vi "template.created_at.vi"(8 "error in":errorcluster, 11 "Template in":refnum<class "Template.lvclass">) -> (0 "error out":errorcluster, 3 "Template out":refnum<class "Template.lvclass">)   [LabVIEW 2020, in "Template.lvclass"]
doc: "Returns the time the template was created."
uses:
  Template.lvclass
  Template.lvclass/Template.ctl
  client.lvlib
panel:
  out "out_millis out":dbl
  in  "out_millis":dbl
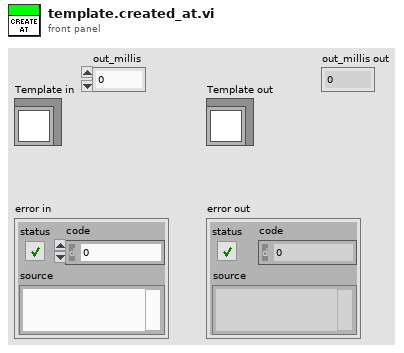
[diagram p1: front panel]
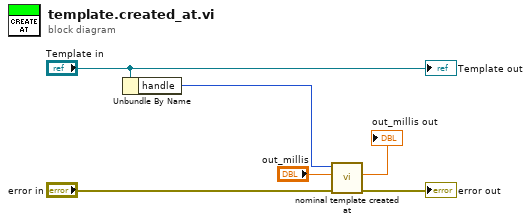
[diagram p0: block diagram]
diagram:
  n1 = Unbundle By Name("Template in") -> ("handle"=w4:i32)
  n2 = call "nominal template created at.vi"("error in (no error)"="error in", "out_millis"="out_millis", "template_"=w4) -> ("error out"=→"error out":errorcluster, "out_millis out"=→"out_millis out":dbl)  [unwired: 6 in, 1 out]
  "Template out" <- "Template in"
